vi "Generate Histogram Data.vi"(1 "noise level":dbl=1.0 format="%0.2f", 2 "number of points":i32=100) -> (0 "Histogram":dbl[](graph))   [LabVIEW 2013]
uses:
  <vilib>/Analysis/NI_AALBase.lvlib
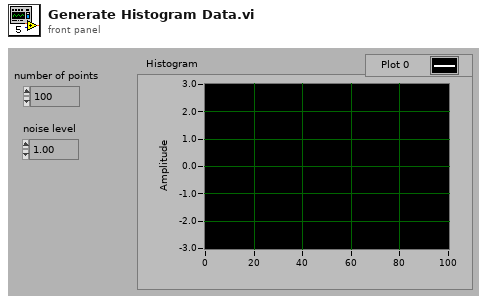
[diagram p1: front panel]
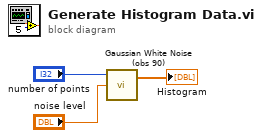
[diagram p0: block diagram]
diagram:
  n1 = call <vilib>:"Gaussian White Noise (obs 90).vi"("standard deviation"="noise level", "samples"="number of points") -> ("Gaussian noise pattern"=→"Histogram":dbl[])  [unwired: 1 in, 1 out]
